vi "Replace Attribute Value.vi"(8 "error in (no error)":errorcluster, 9 "New Value":string, 10 "Attribute Name":string, 11 "node in":refnum<k20>) -> (0 "error out":errorcluster, 3 "Node Out":refnum<k20>)   [LabVIEW 2019, in "ParseSVG.lvclass"]
uses:
  ParseSVG.lvclass
  <vilib>/xml/Close Reference(NNMap).vi
  <vilib>/xml/Close Reference(Node).vi
  <resource>/objmgr/DOMUserDefRef.rc
  <vilib>/xml/NI_XML.lvlib
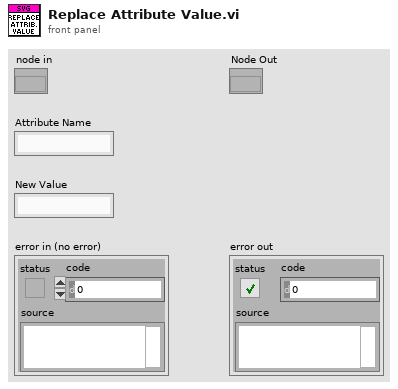
[diagram p1: front panel]
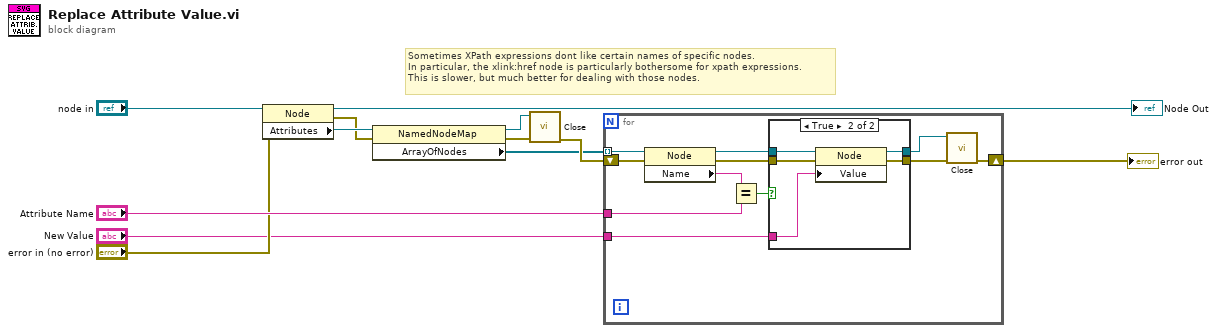
[diagram p0: block diagram]
diagram:
  # "Sometimes XPath expressions dont like certain names of specific nodes. \nIn particular, the xlink:href node is particularly bothersome for xpath expressions. \nThis is slower, but much better for dealing with those nodes."
  n1 = property class="Node"(reference="node in", error in="error in (no error)") -> (reference out=→"Node Out":refnum<k20>, error out=w9:errorcluster, "Attributes"=w11:refnum<k20>)
  n2 = property class="NamedNodeMap"(reference=w11, error in=w9) -> (reference out=w7:refnum<k20>, error out=w10:errorcluster, "ArrayOfNodes"=w6:refnum<k20>[])
  n3 = call-poly <vilib>:"Close.vi"("error in (no error)"=w10, "named node map"=w7) -> ("error out"=w8:errorcluster)  [unwired: 7 in]
  n4 = for {
    tunnel: w6 -> [w23] mode=indexing
    tunnel: "Attribute Name" -> [w15]
    shift-right: [w21] -> w1
    shift-left: w8 -> [w22]
    tunnel: "New Value" -> [w14]
    n5 = property class="Node"(reference=w23, error in=w22) -> (reference out=w17:refnum<k20>, error out=w20:errorcluster, "Name"=w16:string)
    n6 = Equal?(x=w16, y=w15) -> (x = y?=w13:bool)
    n7 = case shown="True" w13 {
      tunnel: w20 -> [w24 w30]
      tunnel: [w24 w29] -> w19
      tunnel: [w25 w28] -> w18
      tunnel: w17 -> [w25 w27]
      tunnel: w14 -> [_ w26]
      frame False {
      }
      frame True {
        n8 = property class="Node"(reference=w27, error in=w30, "Value"=w26) -> (reference out=w28:refnum<k20>, error out=w29:errorcluster)
      }
    }
    n9 = call-poly <vilib>:"Close.vi"("error in (no error)"=w19, "node"=w18) -> ("error out"=w21:errorcluster)  [unwired: 7 in]
  }
  "error out" <- w1
